vi "recibe_firebase_json.vi"() -> ()   [LabVIEW 2025]
uses:
  <vilib>/httpClient/LabVIEWHTTPClient.lvlib
panel:
  out "Rele":bool
  out "Hora":string
  out "Fecha":string
  out "Accionamiento":dbl
  in  "stop":bool
  out "error out":errorcluster
  out "body":string
  out "headers":string
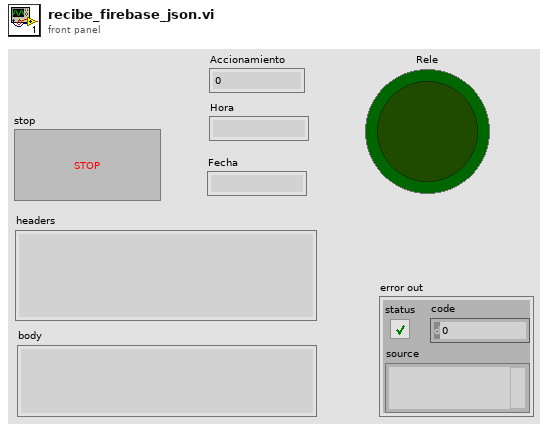
[diagram p1: front panel]
types:
  T1 = cluster{"Accionamiento":dbl, "Fecha":string, "Hora":string, "Rele":bool}
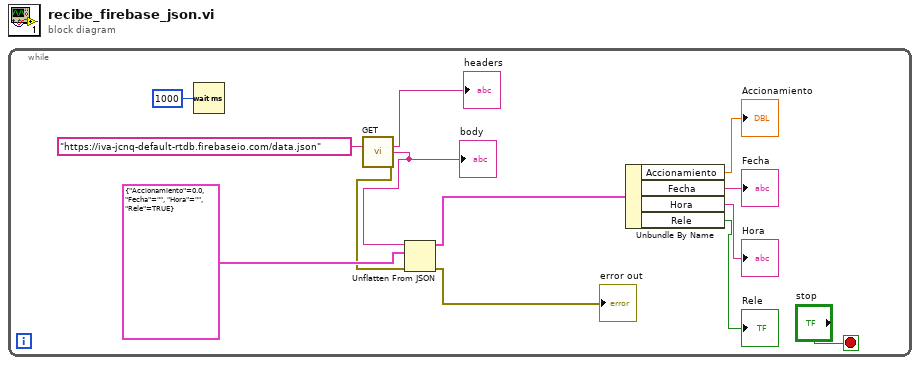
[diagram p0: block diagram]
diagram:
  n1 = while {
    stop <- "stop" stop-if-true
    n2 = Wait (ms)(milliseconds to wait=u32 1000) -> ()  [unwired: 1 out]
    n3 = call <vilib>:"GET.vi"("url"="https://iva-jcnq-default-rtdb.firebaseio.com/data.json") -> ("headers"=→"headers":string, "body"=w4:string, "error out"=w3:errorcluster)  [unwired: 11 in, 1 out]
    "body" <- w4
    n4 = Unflatten From JSON(JSON string=w4, type and defaults=T1 {"Accionamiento"=0.0, "Fecha"="", "Hora"="", "Rele"=TRUE}, error in (no error)=w3) -> (value=w1:T1, error out=→"error out":errorcluster)  [unwired: 4 in]
    n5 = Unbundle By Name(w1) -> ("Accionamiento"=→"Accionamiento":dbl, "Fecha"=→"Fecha":string, "Hora"=→"Hora":string, "Rele"=→"Rele":bool)
  }
